vi "Receive FC2 ILC Inputs.vi"(8 "error in (no error)":errorcluster, 11 "Model in":refnum<class "Model.lvclass">) -> (0 "error out":errorcluster, 3 "Model out":refnum<class "Model.lvclass">)   [LabVIEW 2015, in "Model.lvclass"]
uses:
  Model.lvclass
  Model.lvclass/Model.ctl
  <userlib>/Common/ILC/ILC/ILC.lvclass
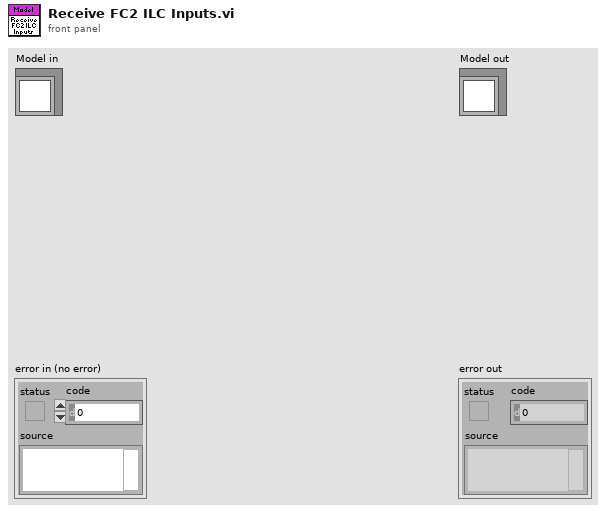
[diagram p1: front panel]
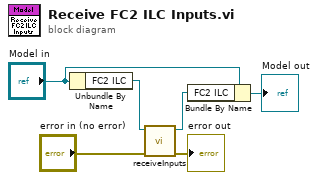
[diagram p0: block diagram]
diagram:
  n1 = Unbundle By Name("Model in") -> ("FC2 ILC"=w2:refnum<class "ILC.lvclass">)
  n2 = call <userlib>:"receiveInputs.vi"("error in (no error)"="error in (no error)", "ILC in"=w2) -> ("error out"=→"error out":errorcluster, "ILC out"=w1:refnum<class "ILC.lvclass">)  [unwired: 6 in, 2 out]
  n3 = Bundle By Name(cluster="Model in", "FC2 ILC"=w1) -> (→"Model out":refnum<class "Model.lvclass">)
